vi "IO_Set Status Color.vi"(8 "Colors [4] in":cluster{u32, u32}[](array[cluster]), 11 "Bench Status":T1) -> ()   [LabVIEW 2024]
uses:
  Control Definitions/Def Bench Status.ctl
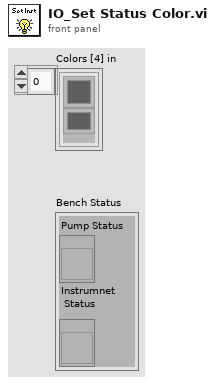
[diagram p1: front panel]
types:
  T1 = typedef "Def Bench Status.ctl" = cluster{"Pump Status":refnum<vi>, "Instrumnet\n Status":refnum<vi>}
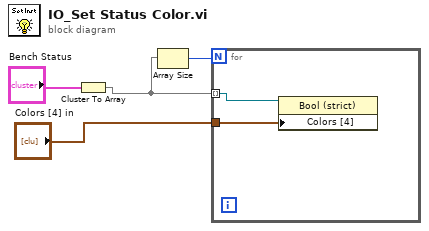
[diagram p0: block diagram]
diagram:
  n1 = Cluster To Array(cluster="Bench Status") -> (array=w1:refnum<vi>[])
  n2 = Array Size(array=w1) -> (size(s)=w2:i32)
  n3 = for {
    N: w2 -> [_]
    tunnel: "Colors [4] in" -> [w6]
    tunnel: w1 -> [w5] mode=indexing
    n4 = property class="Bool (strict)"(reference=w5, "Colors [4]"=w6) -> ()  [unwired: 1 in, 2 out]
  }
